vi "Configure Trigger (Setup or Hold).vi"(0 "VISA resource name":refnum<visa-resource-name>, 1 "Data Source (1: Channel 1)":u16(ring)=1 items=["Channel 1"=1, "Channel 2"=2, "Channel 3"=3, "Channel 4"=4], 2 "Low Threshold (0.001 V)":dbl=0.001, 3 "High Threshold (0.01 V)":dbl=0.01, 5 "Mode (0: Setup)":u16(ring) items=["Setup", "Hold", "Setup And Hold"], 7 "Setup Time (1.5e-9 V)":dbl=1.5e-09, 9 "Hold Time (1.5e-9 V)":dbl=1.5e-09, 11 "error in (no error)":errorcluster, 12 "Clock Source (2: Channel 2)":u16(ring)=2 items=["Channel 1"=1, "Channel 2"=2, "Channel 3"=3, "Channel 4"=4], 13 "Clock Level (0.0 V)":dbl, 14 "Clock Polarity (0: Positive)":u16(ring) items=["Positive", "Negative"]) -> (4 "VISA resource name out":refnum<visa-resource-name>, 15 "error out":errorcluster)   [LabVIEW 2012, in "Agilent 8000 Series.lvlib"]
doc: "Configures the setup and hold time violation trigger. It configures Mode, Setup Time Hold Time, Data Source and Clock Source properties."
uses:
  Agilent 8000 Series.lvlib
panel:
  # "Data"
  # "Clock"
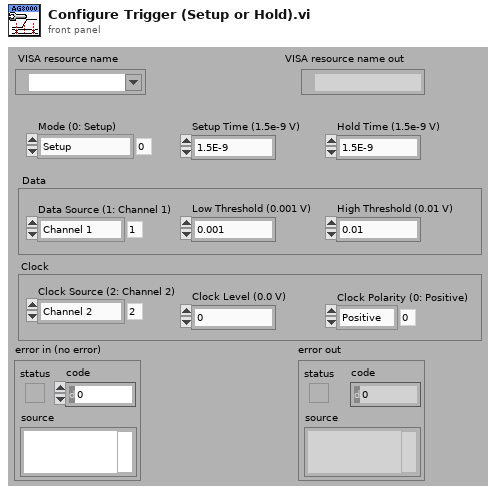
[diagram p1: front panel]
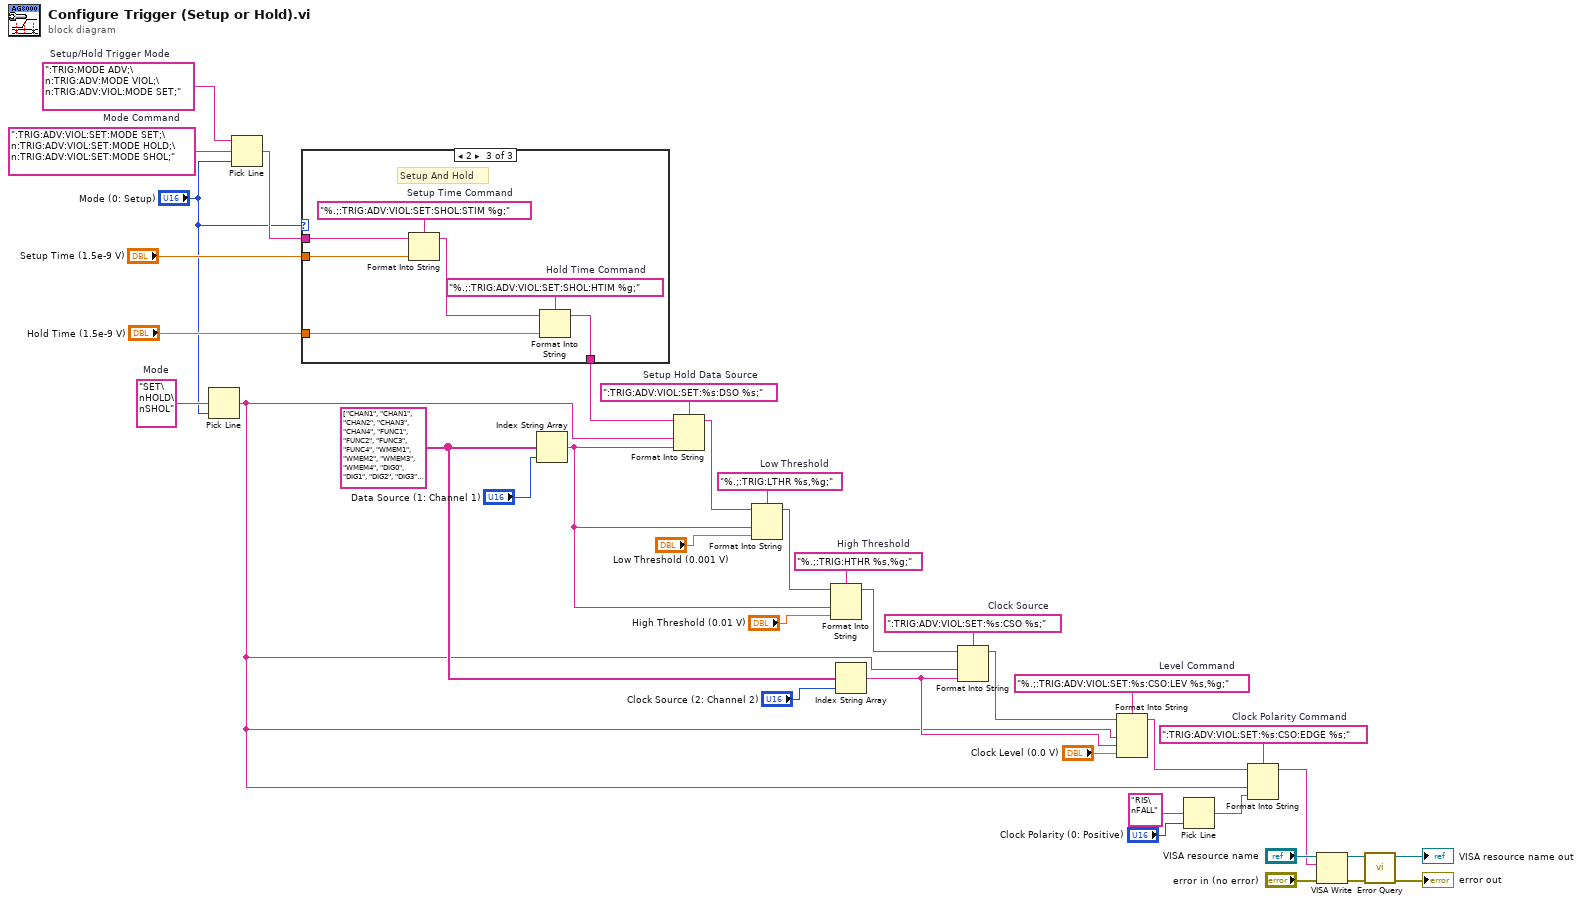
[diagram p0: block diagram]
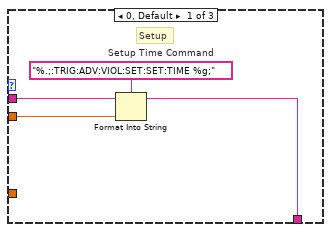
[diagram p2: hidden frame]
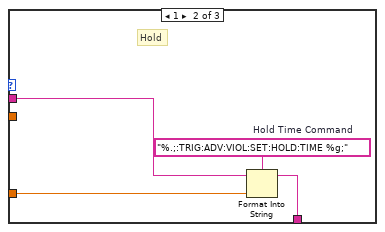
[diagram p3: hidden frame]
diagram:
  w5 = ":TRIG:ADV:VIOL:SET:%s:CSO:EDGE %s;"  # Clock Polarity Command
  w11 = "%.;:TRIG:ADV:VIOL:SET:%s:CSO:LEV %s,%g;"  # Level Command
  w13 = ":TRIG:ADV:VIOL:SET:%s:CSO %s;"  # Clock Source
  w19 = "%.;:TRIG:HTHR %s,%g;"  # High Threshold
  w21 = "%.;:TRIG:LTHR %s,%g;"  # Low Threshold
  w23 = ":TRIG:ADV:VIOL:SET:%s:DSO %s;"  # Setup Hold Data Source
  w26 = "SET\nHOLD\nSHOL"  # Mode
  w14 = string[] ["CHAN1", "CHAN1", "CHAN2", "CHAN3", "CHAN4", "FUNC1", "FUNC2", "FUNC3", "FUNC4", "WMEM1", "WMEM2", "WMEM3", "WMEM4", "DIG0", "DIG1", "DIG2", "DIG3", "DIG4", "DIG5", "DIG6", "DIG7", "DIG8", "DIG9", "DIG10", "DIG11", "DIG12", "DIG13", "DIG14", "DIG15", "AUX", "LINE"]
  w32 = ":TRIG:ADV:VIOL:SET:MODE SET;\n:TRIG:ADV:VIOL:SET:MODE HOLD;\n:TRIG:ADV:VIOL:SET:MODE SHOL;"  # Mode Command
  w31 = ":TRIG:MODE ADV;\n:TRIG:ADV:MODE VIOL;\n:TRIG:ADV:VIOL:MODE SET;"  # Setup/Hold Trigger Mode
  n1 = Pick Line(multi-line string=w26, line index="Mode (0: Setup)") -> (output string=w2:string)  [unwired: 1 in]
  n2 = Pick Line(string ("")=w31, multi-line string=w32, line index="Mode (0: Setup)") -> (output string=w29:string)
  n3 = case shown="2" "Mode (0: Setup)" {
    tunnel: "Setup Time (1.5e-9 V)" -> [w41 _ w52]
    tunnel: w29 -> [w40 w44 w51]
    tunnel: "Hold Time (1.5e-9 V)" -> [_ w45 w48]
    tunnel: [w39 w43 w47] -> w24
    frame 0, Default {
      w42 = "%.;:TRIG:ADV:VIOL:SET:SET:TIME %g;"  # Setup Time Command
      # "Setup"
      n4 = Format Into String(format string=w42, initial string=w40, w41) -> (resulting string=w39:string)  [unwired: 1 in, 1 out]
    }
    frame 1 {
      w46 = "%.;:TRIG:ADV:VIOL:SET:HOLD:TIME %g;"  # Hold Time Command
      # "Hold"
      n5 = Format Into String(format string=w46, initial string=w44, w45) -> (resulting string=w43:string)  [unwired: 1 in, 1 out]
    }
    frame 2 {
      w50 = "%.;:TRIG:ADV:VIOL:SET:SHOL:HTIM %g;"  # Hold Time Command
      w53 = "%.;:TRIG:ADV:VIOL:SET:SHOL:STIM %g;"  # Setup Time Command
      # "Setup And Hold"
      n6 = Format Into String(format string=w53, initial string=w51, w52) -> (resulting string=w49:string)  [unwired: 1 in, 1 out]
      n7 = Format Into String(format string=w50, initial string=w49, w48) -> (resulting string=w47:string)  [unwired: 1 in, 1 out]
    }
  }
  n8 = Index String Array(1:"Data Source (1: Channel 1)", 2:w14) -> (0:w17:string)  [unwired: 1 in]
  n9 = Format Into String(format string=w23, initial string=w24, w2, w17) -> (resulting string=w22:string)  [unwired: 1 in, 1 out]
  n10 = Format Into String(format string=w21, initial string=w22, w17, "Low Threshold (0.001 V)") -> (resulting string=w18:string)  [unwired: 1 in, 1 out]
  n11 = Format Into String(format string=w19, initial string=w18, w17, "High Threshold (0.01 V)") -> (resulting string=w12:string)  [unwired: 1 in, 1 out]
  n12 = Index String Array(1:"Clock Source (2: Channel 2)", 2:w14) -> (0:w8:string)  [unwired: 1 in]
  n13 = Format Into String(format string=w13, initial string=w12, w2, w8) -> (resulting string=w10:string)  [unwired: 1 in, 1 out]
  n14 = Format Into String(format string=w11, initial string=w10, w2, w8, "Clock Level (0.0 V)") -> (resulting string=w4:string)  [unwired: 1 in, 1 out]
  n15 = Pick Line(multi-line string="RIS\nFALL" ("string (\"\")"), line index="Clock Polarity (0: Positive)") -> (output string=w3:string)  [unwired: 1 in]
  n16 = Format Into String(format string=w5, initial string=w4, w2, w3) -> (resulting string=w1:string)  [unwired: 1 in, 1 out]
  n17 = VISA Write(VISA resource name="VISA resource name", write buffer=w1, error in (no error)="error in (no error)") -> (VISA resource name out=w34:refnum<visa-resource-name>, error out=w33:errorcluster)  [unwired: 1 out]
  n18 = call "Error Query.vi"("error in (no error)"=w33, "VISA resource name"=w34) -> ("error out"=→"error out":errorcluster, "VISA resource name out"=→"VISA resource name out":refnum<visa-resource-name>)  [unwired: 6 in, 2 out]
